vi "Mouse In.vi"(8 "error in (no error)":errorcluster, 10 "MousePoint":cluster{"x":i16, "y":i16}, 11 "Triangle in":refnum<class "Triangle.lvclass">) -> (0 "error out":errorcluster, 2 "In?":bool, 3 "Triangle out":refnum<class "Triangle.lvclass">)   [LabVIEW 2015, in "Triangle.lvclass"]
uses:
  Triangle.lvclass
  Graphic/Graphic.lvclass/Graphic.ctl
  Graphic/Graphic.lvclass
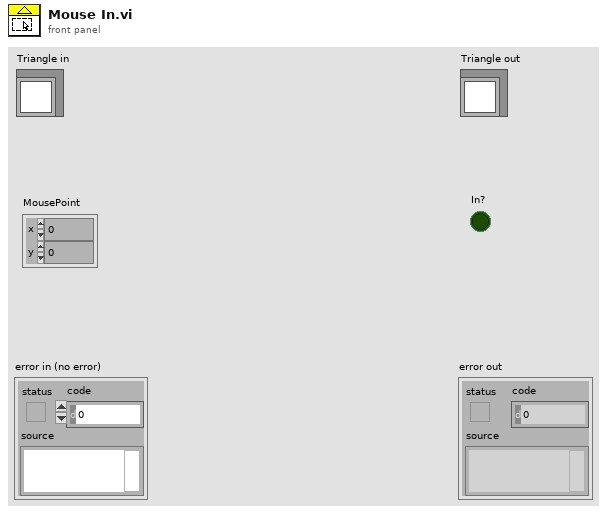
[diagram p1: front panel]
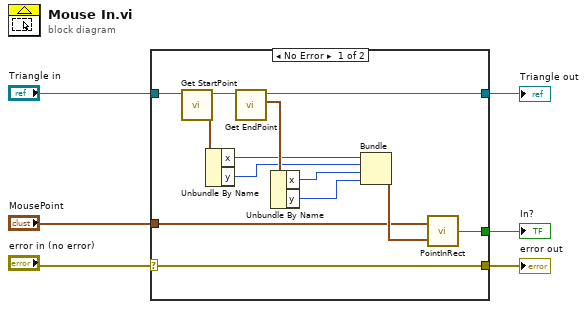
[diagram p0: block diagram]
diagram:
  n1 = case shown="No Error" "error in (no error)" {
    selector: "error in (no error)" -> [w19 w21]
    tunnel: "Triangle in" -> [w18 w20]
    tunnel: [w16 w20] -> w4
    tunnel: "MousePoint" -> [w8 _]
    tunnel: [w7 _] -> w2
    tunnel: [w19 w21] -> w3
    frame No Error {
      n2 = call "Get StartPoint.vi"("Graphic in"=w18) -> ("StartPoint"=w15:cluster{"x":i16, "y":i16}, "Graphic out"=w17:refnum<class "Triangle.lvclass">)  [unwired: 8 in, 1 out]
      n3 = Unbundle By Name(w15) -> ("x"=w13:i16, "y"=w12:i16)
      n4 = call "Get EndPoint.vi"("Graphic in"=w17) -> ("EndPoint"=w14:cluster{"x":i16, "y":i16}, "Graphic out"=w16:refnum<class "Triangle.lvclass">)  [unwired: 8 in, 1 out]
      n5 = Unbundle By Name(w14) -> ("x"=w11:i16, "y"=w10:i16)
      n6 = Bundle("x"=w13, "y"=w12, "x"=w11, "y"=w10) -> (w9:cluster{"x":i16, "y":i16, "x":i16, "y":i16})  [unwired: 1 in]
      n7 = call <vilib>:"PointInRect.vi"("rect"=w9, "point"=w8) -> ("pt in rect"=w7:bool)
    }
    frame Error {
    }
  }
  "error out" <- w3
  "Triangle out" <- w4
  "In?" <- w2
